vi "Set_4G_UL_Frequency.vi"(8 "error in (no error)":errorcluster, 10 "value":i32=1748 max=503, 11 "Base Station":T1) -> (0 "error out":errorcluster, 3 "Output String":string)   [LabVIEW 2021]
uses:
  Controls/Base_Station_Emulator.ctl
  Controls/TCP_FGV.ctl
panel:
  # "<value> specifies the uplink frequency, in MHz. The possible values are from 1920 to 1980 for band 1, 1850 to 1910 for band 2, 1710 to 1785 for band 3,  1710 to 1755 for band 4,\n  824 to 849 for band 5, 830 to 840 for band 6, 2500 to 2570 for band 7, 880 to 915 for band 8,  1749.9 to 1784.9 for band 19, \n832 to 862 for band 20, 814 to 849  for band 26 and 2300 to 2400 for band 40.\nThe default value is 1747.5."
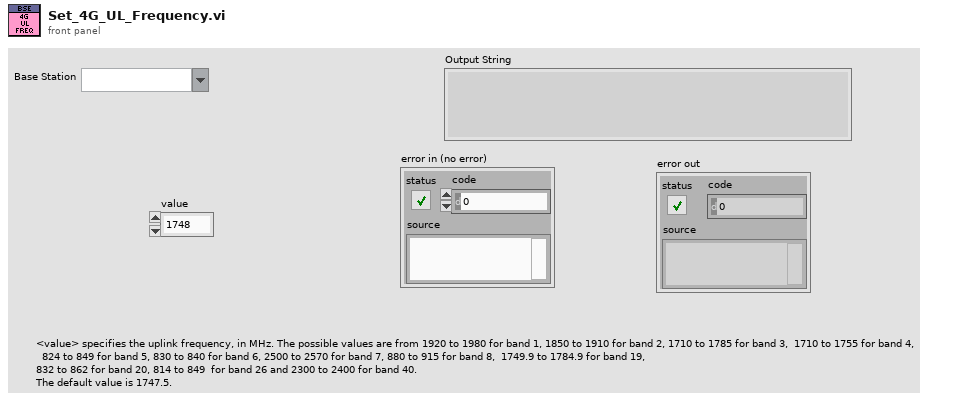
[diagram p1: front panel]
types:
  T1 = typedef "Base_Station_Emulator.ctl" = string
  T2 = typedef "TCP_FGV.ctl" = enum16{"Open", "Read", "Write", "Close"}
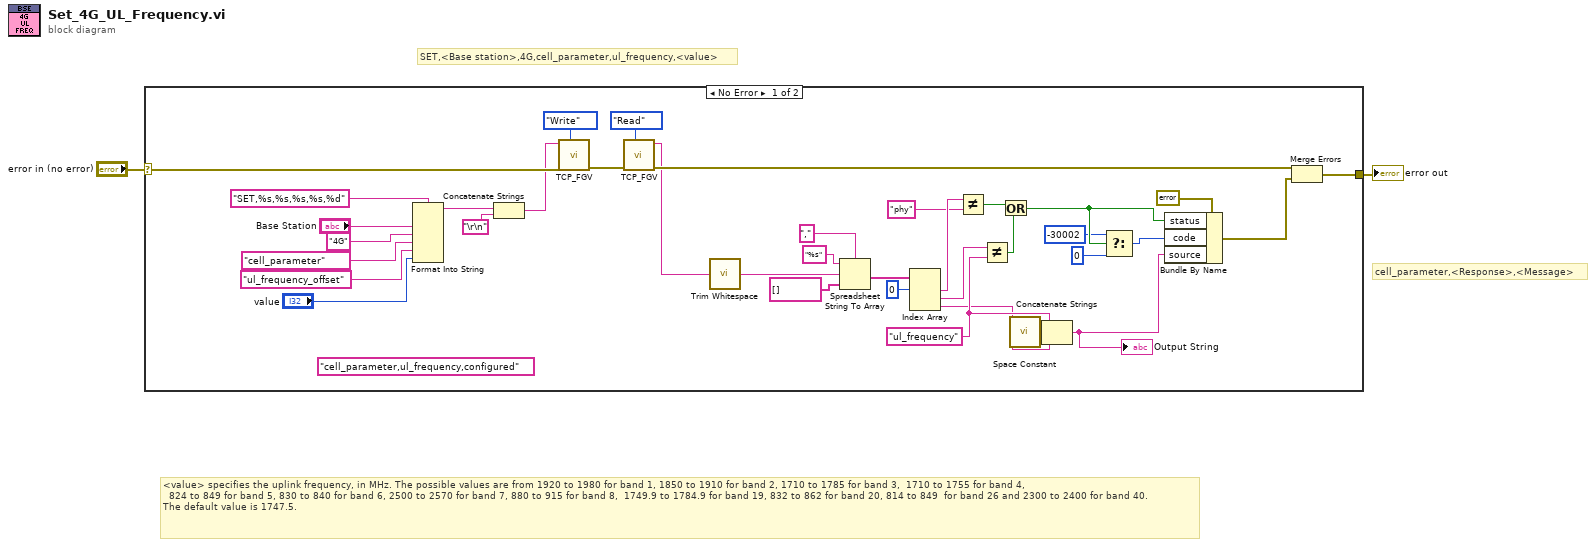
[diagram p0: block diagram]
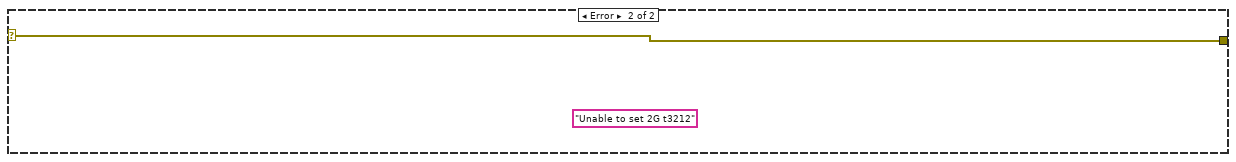
[diagram p2: hidden frame]
diagram:
  # "<value> specifies the uplink frequency, in MHz. The possible values are from 1920 to 1980 for band 1, 1850 to 1910 for band 2, 1710 to 1785 for band 3,  1710 to 1755 for band 4,\n  824 to 849 for band 5, 830 to 840 for band 6, 2500 to 2570 for band 7, 880 to 915 for band 8,  1749.9 to 1784.9 for band 19, 832 to 862 for band 20, 814 to 849  for band 26 and 2300 to 2400 for band 40.\nThe default value is 1747.5."
  # "SET,<Base station>,4G,cell_parameter,ul_frequency,<value>"
  # "cell_parameter,<Response>,<Message>"
  n1 = case shown="No Error" "error in (no error)" {
    selector: "error in (no error)" -> [w36 w40]
    tunnel: [w14 w40] -> w1
    frame No Error {
      (unwired) "cell_parameter,ul_frequency,configured" ("format string")
      w12 = "ul_frequency"
      n2 = Format Into String(format string="SET,%s,%s,%s,%s,%d", "Base Station", "4G", "cell_parameter", "ul_frequency_offset", "value") -> (resulting string=w6:string)  [unwired: 2 in, 1 out]
      n3 = Concatenate Strings(w6, "\r\n") -> (w5:string)
      n4 = call "TCP_FGV.vi"("Command"=w5, "error in (no error)"=w36, "Operation"=TCP_FGV."Write") -> ("error out"=w15:errorcluster)  [unwired: 6 in, 1 out]
      n5 = call "TCP_FGV.vi"("error in (no error)"=w15, "Operation"=TCP_FGV."Read") -> ("Data Out"=w4:string, "error out"=w17:errorcluster)  [unwired: 7 in]
      n6 = call <vilib>:"Trim Whitespace.vi"("string"=w4) -> ("trimmed string"=w31:string)  [unwired: 1 in]
      n7 = Spreadsheet String To Array(delimiter (Tab)=",", format string="%s", spreadsheet string=w31, array type (2D Dbl)=string[] []) -> (array=w27:string[])
      n8 = Index Array(array=w27, index #1=0 ("index")) -> (element #1=w28:string, element #2=w18:string, element #3=w11:string)  [unwired: 2 in]
      n9 = Not Equal?(x=w28, y="phy" ("format string")) -> (x != y?=w29:bool)
      n10 = Not Equal?(x=w18, y=w12) -> (x != y?=w30:bool)
      n11 = Or(x=w29, y=w30) -> (x .or. y?=w32:bool)
      n12 = call <vilib>:"Space Constant.vi"() -> ("String"=w13:string)
      n13 = Concatenate Strings(w12, w13, w11) -> (w10:string)
      "Output String" <- w10
      n14 = Select(t=-30002 ("code"), s=w32, f=0 ("code")) -> (s? t:f=w33:i32)
      n15 = Bundle By Name(cluster=errorcluster {"status"=FALSE, "code"=0, "source"=""} ("error constant"), "status"=w32, "code"=w33, "source"=w10) -> (w16:errorcluster)
      n16 = Merge Errors(w17, w16) -> (w14:errorcluster)
    }
    frame Error {
      (unwired) "Unable to set 2G t3212" ("source")
    }
  }
  "error out" <- w1
